vi "ini_objects_parse.vi"(8 "error in":errorcluster, 11 "items command":string="d;btn ok;[setup];btn_ok;\n;settle [ms];[setup];settle\n\n;btn ok;[setup];btn_ok\n;settle [ms];[setup];settle") -> (0 "error out":errorcluster, 3 "ini items":T1[](array[typedef]))   [LabVIEW 2018]
uses:
  ini_parse_row.ctl
  <vilib>/regexp/Match Regular Expression.xnode
panel:
  out "Array":string[](array[string])
  # "Examples:\nvi path;my cluster->object in cluster;ini section;ini key;ini default value (optional)\nvi path;my object;ini section;ini key;ini default value (optional)"
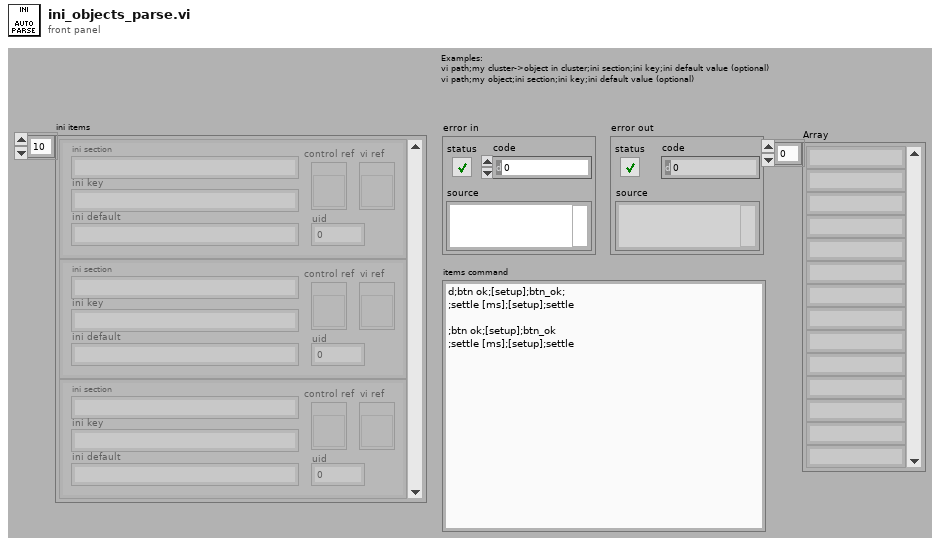
[diagram p1: front panel]
types:
  T1 = typedef "ini_parse_row.ctl" = cluster{"ini section":string, "ini key":string, "ini default":string, "control ref":refnum<vi>, "uid":i32, "vi ref":refnum<vi>}
  T2 = cluster{"[0]":string, "[1]":string, "[2]":string, "[3]":string, "[4]":string}
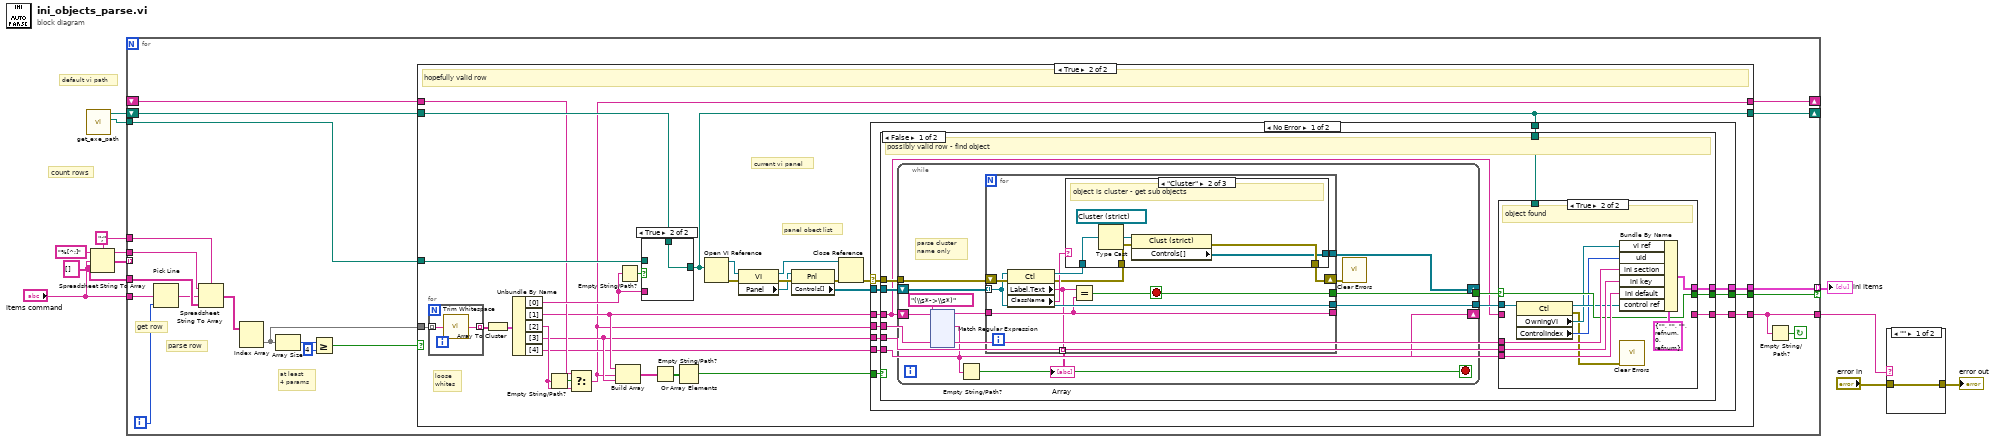
[diagram p0: block diagram]
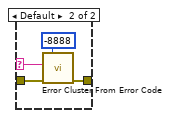
[diagram p2: hidden frame]
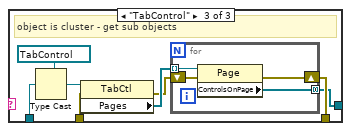
[diagram p5: hidden frame]
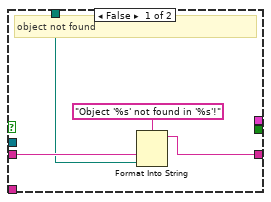
[diagram p6: hidden frame]
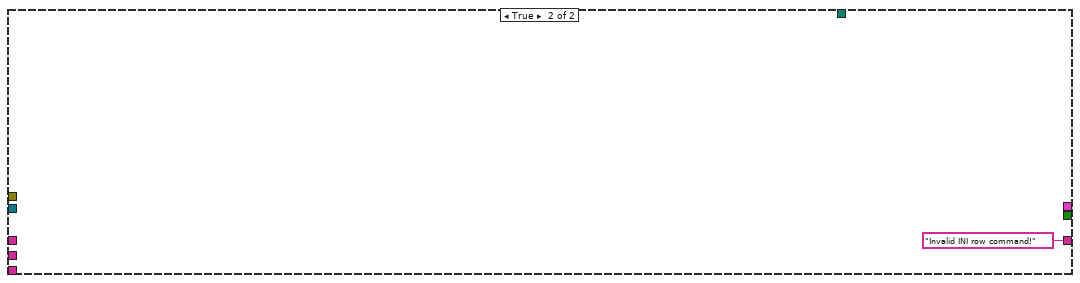
[diagram p7: hidden frame]
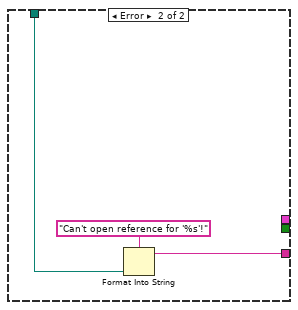
[diagram p8: hidden frame]
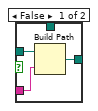
[diagram p9: hidden frame]
diagram:
  w9 = ";" ("delimiter (Tab)")
  w8 = string[][] []
  w7 = "%[^;]" ("format string")
  # "default vi path"
  # "count rows"
  n1 = call "get_exe_path.vi"() -> ("application root path"=w1:path, "full path"=w6:path)  [unwired: 2 out]
  n2 = Spreadsheet String To Array(delimiter (Tab)=w9, format string=w7, spreadsheet string="items command", array type (2D Dbl)=w8) -> (array=w11:string[][])
  n3 = for {
    tunnel: w11 -> [_] mode=indexing
    tunnel: "items command" -> [w31]
    tunnel: w9 -> [w29]
    tunnel: w8 -> [w28]
    tunnel: w7 -> [w26]
    tunnel: w1 -> [w21]
    shift-right: [w20] -> _
    shift-left: w6 -> [w19]
    shift-right: [w17] -> _
    shift-left: _ -> [w18]
    tunnel: [w15] -> w2 mode=indexing if=w14
    tunnel: [w13] -> w3
    i -> [w30]
    stop <- w12 continue-if-true
    # "at least\n4 params"
    # "parse row"
    # "get row"
    n4 = Pick Line(multi-line string=w31, line index=w30) -> (output string=w27:string)  [unwired: 1 in]
    n5 = Spreadsheet String To Array(delimiter (Tab)=w29, format string=w26, spreadsheet string=w27, array type (2D Dbl)=w28) -> (array=w25:string[][])
    n6 = Index Array(array=w25) -> (element=w16:string[])  [unwired: 2 in]
    n7 = Array Size(array=w16) -> (size(s)=w24:i32)
    n8 = Greater Or Equal?(x=w24, y=4) -> (x >= y?=w22:bool)
    n9 = case shown="True" w22 {
      tunnel: w16 -> [_ w62]
      tunnel: w21 -> [_ w57]
      tunnel: [w33 w36] -> w20
      tunnel: w19 -> [w33 w56]
      tunnel: w18 -> [w32 w46]
      tunnel: [w32 w34] -> w17
      tunnel: [_ w38] -> w15
      tunnel: [_ w37] -> w14
      tunnel: [_ w35] -> w13
      frame False {
      }
      frame True {
        # "panel obect list"
        # "current vi panel"
        # "loose\nwhites"
        # "hopefully valid row"
        n10 = for {
          tunnel: w62 -> [w267] mode=indexing
          tunnel: [w266] -> w61 mode=indexing
          n11 = call <vilib>:"Trim Whitespace.vi"("string"=w267) -> ("trimmed string"=w266:string)  [unwired: 1 in]
        }
        n12 = Array To Cluster(array=w61) -> (cluster=w60:T2)
        n13 = Unbundle By Name(w60) -> ("[0]"=w58:string, "[1]"=w42:string, "[2]"=w41:string, "[3]"=w40:string, "[4]"=w39:string)
        n14 = Empty String/Path?(string/path=w41) -> (empty?=w47:bool)
        n15 = Select(t=w46, s=w47, f=w41) -> (s? t:f=w34:string)
        n16 = Build Array(w42, w34, w40) -> (w45:string[])
        n17 = Empty String/Path?(string/path=w58) -> (empty?=w59:bool)
        n18 = case shown="True" w59 {
          tunnel: w58 -> [w263 _]
          tunnel: w57 -> [w264 _]
          tunnel: [w262 w265] -> w36
          tunnel: w56 -> [_ w265]
          frame False {
            n19 = Build Path(base path=w264, name or relative path=w263) -> (appended path=w262:path)
          }
          frame True {
          }
        }
        n20 = Empty String/Path?(string/path=w45) -> (empty?=w44:bool[])
        n21 = Or Array Elements(Boolean array=w44) -> (logical OR=w43:bool)
        n22 = Open VI Reference(vi path=w36) -> (vi reference=w54:refnum<vi>, error out=w55:errorcluster)  [unwired: 5 in]
        n23 = property class="VI"(reference=w54, error in=w55) -> (reference out=w50:refnum<vi>, error out=w53:errorcluster, "Panel"=w52:refnum<vi>)
        n24 = property class="Pnl"(reference=w52, error in=w53) -> (error out=w51:errorcluster, "Controls[]"=w48:refnum<vi>[])  [unwired: 1 out]
        n25 = Close Reference(reference=w50, error in (no error)=w51) -> (error out=w49:errorcluster)
        n26 = case shown="No Error" w49 {
          selector: w49 -> [w72 _]
          tunnel: w48 -> [w71 _]
          tunnel: w43 -> [w73 _]
          tunnel: w42 -> [w70 _]
          tunnel: w34 -> [w69 _]
          tunnel: w40 -> [w68 _]
          tunnel: w39 -> [w67 _]
          tunnel: [w66 _] -> w38
          tunnel: [w65 _] -> w37
          tunnel: w36 -> [w64 w259]
          tunnel: [w63 w260] -> w35
          frame No Error {
            n27 = case shown="False" w73 {
              tunnel: w72 -> [w85 _]
              tunnel: w71 -> [w84 _]
              tunnel: w70 -> [w74 _]
              tunnel: w69 -> [w81 _]
              tunnel: w68 -> [w80 _]
              tunnel: w67 -> [w79 _]
              tunnel: [w78 _] -> w66
              tunnel: [w77 _] -> w65
              tunnel: w64 -> [w76 _]
              tunnel: [w75 "Invalid INI row command!"] -> w63
              frame False {
                # "possibly valid row - find object"
                n28 = while {
                  tunnel: w85 -> [w97]
                  tunnel: [w96] -> w83
                  tunnel: [w94] -> w82
                  shift-right: [w90] -> _
                  shift-left: w74 -> [w92]
                  shift-right: [w88] -> _
                  shift-left: w84 -> [w87]
                  stop <- w91 stop-if-true
                  # "parse cluster\nname only"
                  n29 = xnode "Match Regular Expression"("input string"=w92, "regular expression"="(\\s*->\\s*)") -> ("before match"=w89:string, "after match"=w90:string)  [unwired: 4 in, 4 out]
                  n30 = Empty String/Path?(string/path=w90) -> (empty?=w91:bool)
                  n31 = for {
                    shift-right: [w216] -> w95
                    shift-left: w97 -> [w223]
                    tunnel: w87 -> [w222] mode=indexing
                    tunnel: w89 -> [w220]
                    tunnel: [w222] -> w94
                    tunnel: [w221] -> w96
                    tunnel: [w220] -> _
                    tunnel: [w215] -> w88
                    tunnel: [w214] -> w86 mode=indexing
                    stop <- w221 stop-if-true
                    n32 = property class="Ctl"(reference=w222, error in=w223) -> (reference out=w219:refnum<vi>, error out=w217:errorcluster, "Label.Text"=w214:string, "ClassName"=w218:string)
                    n33 = case shown="\"Cluster\"" w218 {
                      tunnel: w219 -> [_ w230 w238]
                      tunnel: w217 -> [w224 w227 w235]
                      tunnel: [w224 w226 w232] -> w216
                      tunnel: [_ w225 w231] -> w215
                      frame Default {
                        # "not a cluster"
                      }
                      frame "Cluster" {
                        # "object is cluster - get sub objects"
                        n34 = Type Cast(type=refnum<vi> refnum ("reference"), x=w230) -> (*(type *) &x=w228:refnum<vi>)
                        n35 = property class="Clust (strict)"(reference=w228, error in=w227) -> (error out=w226:errorcluster, "Controls[]"=w225:refnum<vi>[])  [unwired: 1 out]
                      }
                      frame "TabControl" {
                        # "object is cluster - get sub objects"
                        n36 = Type Cast(type=refnum<vi> refnum ("reference"), x=w238) -> (*(type *) &x=w236:refnum<vi>)
                        n37 = property class="TabCtl"(reference=w236, error in=w235) -> (error out=w233:errorcluster, "Pages"=w234:refnum<vi>[])  [unwired: 1 out]
                        n38 = for {
                          tunnel: w234 -> [w242] mode=indexing
                          shift-right: [w239] -> w232
                          shift-left: w233 -> [w241]
                          tunnel: [w240] -> w231 mode=concatenating
                          n39 = property class="Page"(reference=w242, error in=w241) -> (error out=w239:errorcluster, "ControlsOnPage"=w240:refnum<vi>[])  [unwired: 1 out]
                        }
                      }
                    }
                    n40 = Equal?(x=w214, y=w220) -> (x = y?=w221:bool)
                  }
                  "Array" <- w86
                  n41 = call <vilib>:"Clear Errors.vi"("error in (no error)"=w95) -> ()  [unwired: 5 in, 2 out]
                }
                n42 = case shown="True" w83 {
                  selector: w83 -> [_ w252]
                  tunnel: w82 -> [_ w251]
                  tunnel: w81 -> [_ w256]
                  tunnel: w80 -> [_ w255]
                  tunnel: w79 -> [_ w254]
                  tunnel: [_ w253] -> w78
                  tunnel: [_ w252] -> w77
                  tunnel: w74 -> [w245 _]
                  tunnel: w76 -> [w244 _]
                  tunnel: [w243 _] -> w75
                  frame False {
                    # "object not found"
                    n43 = Format Into String(format string="Object '%s' not found in '%s'!", w245, w244) -> (resulting string=w243:string)  [unwired: 2 in, 1 out]
                  }
                  frame True {
                    # "object found"
                    n44 = property class="Ctl"(reference=w251) -> (reference out=w250:refnum<vi>, error out=w247:errorcluster, "OwningVI"=w248:refnum<vi>, "ControlIndex"=w249:i32)  [unwired: 1 in]
                    n45 = Bundle By Name(cluster=T1 {"ini section"="", "ini key"="", "ini default"="", "control ref"=refnum, "uid"=0, "vi ref"=refnum} ("auto ini row"), "vi ref"=w248, "uid"=w249, "ini section"=w256, "ini key"=w255, "ini default"=w254, "control ref"=w250) -> (w253:T1)
                    n46 = call <vilib>:"Clear Errors.vi"("error in (no error)"=w247) -> ()  [unwired: 5 in, 2 out]
                  }
                }
              }
              frame True {
              }
            }
          }
          frame Error {
            n47 = Format Into String(format string="Can't open reference for '%s'!", w259) -> (resulting string=w260:string)  [unwired: 2 in, 1 out]
          }
        }
      }
    }
    n48 = Empty String/Path?(string/path=w13) -> (empty?=w12:bool)
  }
  "ini items" <- w2
  n49 = case shown="\"\"" w3 {
    selector: w3 -> [_ w269]
    tunnel: [w268 w272] -> w5
    tunnel: "error in" -> [w268 w271]
    frame "" {
    }
    frame Default {
      n50 = call <vilib>:"Error Cluster From Error Code.vi"("error in (no error)"=w271, "error message (\"\")"=w269, "error code (0)"=-8888) -> ("error out"=w272:errorcluster)  [unwired: 6 in]
    }
  }
  "error out" <- w5
